vi "EstimateStatorResistance.vi"(11 "motor nameplate information":T1) -> (3 "stator resisitance [ohms]":dbl)   [LabVIEW 2017, in "McsaAnalysisFunctions.lvlib"]
doc: "Regenerates the namplate information for Speed Estimation VI and Torque Load and Efficiency VI and estimates the stator resistance values for air gap torque method based on motor nameplate information."
uses:
  <vilib>/addons/InsightCM/Utilities/Analysis/MCSA/McsaAnalysisFunctions.lvlib
  <vilib>/addons/InsightCM/Utilities/Analysis/MCSA/controls/McsaMotor.ctl
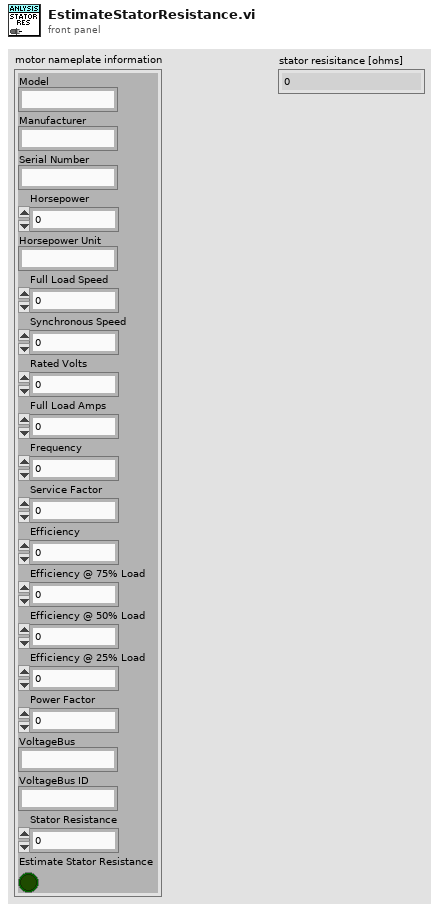
[diagram p1: front panel]
types:
  T1 = typedef "McsaAnalysisFunctions.lvlib/McsaMotor.ctl" = cluster{"Model":string, "Manufacturer":string, "Serial Number":string, "Horsepower":dbl, "Horsepower Unit":string, "Full Load Speed":dbl, "Synchronous Speed":dbl, "Rated Volts":dbl, "Full Load Amps":dbl, "Frequency":dbl, "Service Factor":dbl, "Efficiency":dbl, "Efficiency @ 75% Load":dbl, "Efficiency @ 50% Load":dbl, "Efficiency @ 25% Load":dbl, "Power Factor":dbl, "VoltageBus":string, "VoltageBus ID":string, "Stator Resistance":dbl, "Estimate Stator Resistance":bool}
  T2 = cluster{"synchronous speed [RPM]":dbl, "full load speed [RPM]":dbl, "full load [kW]":dbl, "full load efficiency [%]":dbl, "full load current [A]":dbl}
  T3 = cluster{"synchronous speed [RPM]":dbl, "full load speed [RPM]":dbl, "full load [kW]":dbl, "full load efficiency [%]":dbl, "full load current [A]":dbl}[]
  T4 = cluster{"nominal frequency":enum16{"50 Hz", "60 Hz"}, "motor information":cluster{"synchronous speed [RPM]":dbl, "full load speed [RPM]":dbl, "full load [W]":dbl, "full load efficiency [%]":dbl, "full load current [A]":dbl}[]}
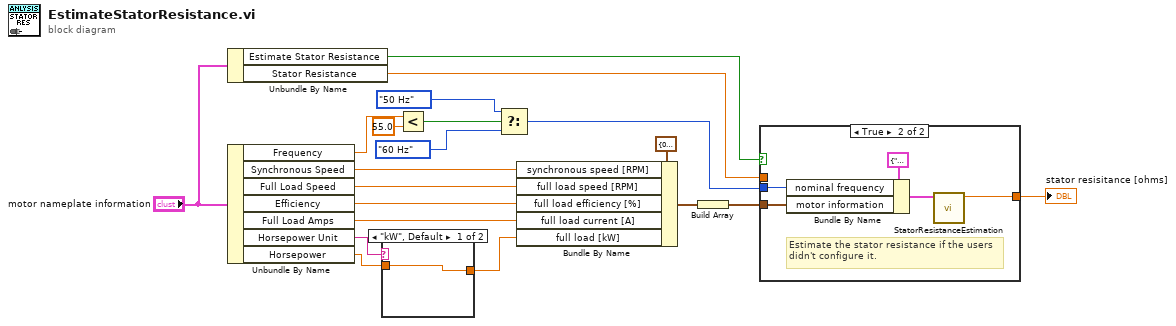
[diagram p0: block diagram]
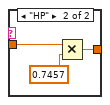
[diagram p3: hidden frame]
diagram:
  n1 = Unbundle By Name("motor nameplate information") -> ("Estimate Stator Resistance"=w3:bool, "Stator Resistance"=w2:dbl)
  n2 = Unbundle By Name("motor nameplate information") -> ("Frequency"=w12:dbl, "Synchronous Speed"=w18:dbl, "Full Load Speed"=w17:dbl, "Efficiency"=w16:dbl, "Full Load Amps"=w15:dbl, "Horsepower Unit"=w7:string, "Horsepower"=w6:dbl)
  n3 = case shown="\"kW\", Default" w7 {
    tunnel: [w21 w23] -> w5
    tunnel: w6 -> [w21 w24]
    frame "kW", Default {
    }
    frame "HP" {
      n4 = Multiply(x=w24, y=0.7457) -> (x*y=w23:dbl)
    }
  }
  n5 = Less?(x=w12, y=55.0) -> (x < y?=w13:bool)
  n6 = Select(t=enum16{"50 Hz", "60 Hz"}."50 Hz" ("nominal frequency"), s=w13, f=enum16{"50 Hz", "60 Hz"}."60 Hz" ("nominal frequency")) -> (s? t:f=w9:enum16{"50 Hz", "60 Hz"})
  n7 = Bundle By Name(cluster=T2 {"synchronous speed [RPM]"=0.0, "full load speed [RPM]"=0.0, "full load [kW]"=0.0, "full load efficiency [%]"=0.0, "full load current [A]"=0.0} ("speed related nameplate data 2"), "synchronous speed [RPM]"=w18, "full load speed [RPM]"=w17, "full load efficiency [%]"=w16, "full load current [A]"=w15, "full load [kW]"=w5) -> (w14:T2)
  n8 = Build Array(w14) -> (w20:T3)
  n9 = case shown="True" w3 {
    tunnel: w20 -> [_ w28]
    tunnel: w9 -> [_ w27]
    tunnel: [w25 w26] -> w1
    tunnel: w2 -> [w25 _]
    frame False {
      # "Utilize the configured value if the\nusers configure it."
    }
    frame True {
      # "Estimate the stator resistance if the users\ndidn't configure it."
      n10 = Bundle By Name(cluster=T4 {"nominal frequency"=enum."50 Hz", "motor information"=[]} ("nameplate information"), "nominal frequency"=w27, "motor information"=w28) -> (w29:T4)
      n11 = call <vilib>:"StatorResistanceEstimation.vi"("nameplate information"=w29) -> ("stator resisitance [ohms]"=w26:dbl)  [unwired: 10 in]
    }
  }
  "stator resisitance [ohms]" <- w1
